vi "DAQ.vi"() -> ()   [LabVIEW 2014]
uses:
  <vilib>/express/express analysis/Spectral/Block/exnSpectralBlock spectral measurements PSD poly.vi
  <vilib>/express/express analysis/Spectral/Block/exnSpectralBlock spectral measurements PSD DDT.vi
  <vilib>/express/express analysis/Spectral/XNode/ExpressSpectralMeasurementsBlockNode.xnode
panel:
  out "Filtered PSD plot":dynamicdata(graph)
  out "RAW PSD plot":dynamicdata(graph)
  out "RAW & filtered Plot":dynamicdata(graph) caption="data"
  in  "File Comment":string caption="Comment"
  in  "Stop Daq":bool
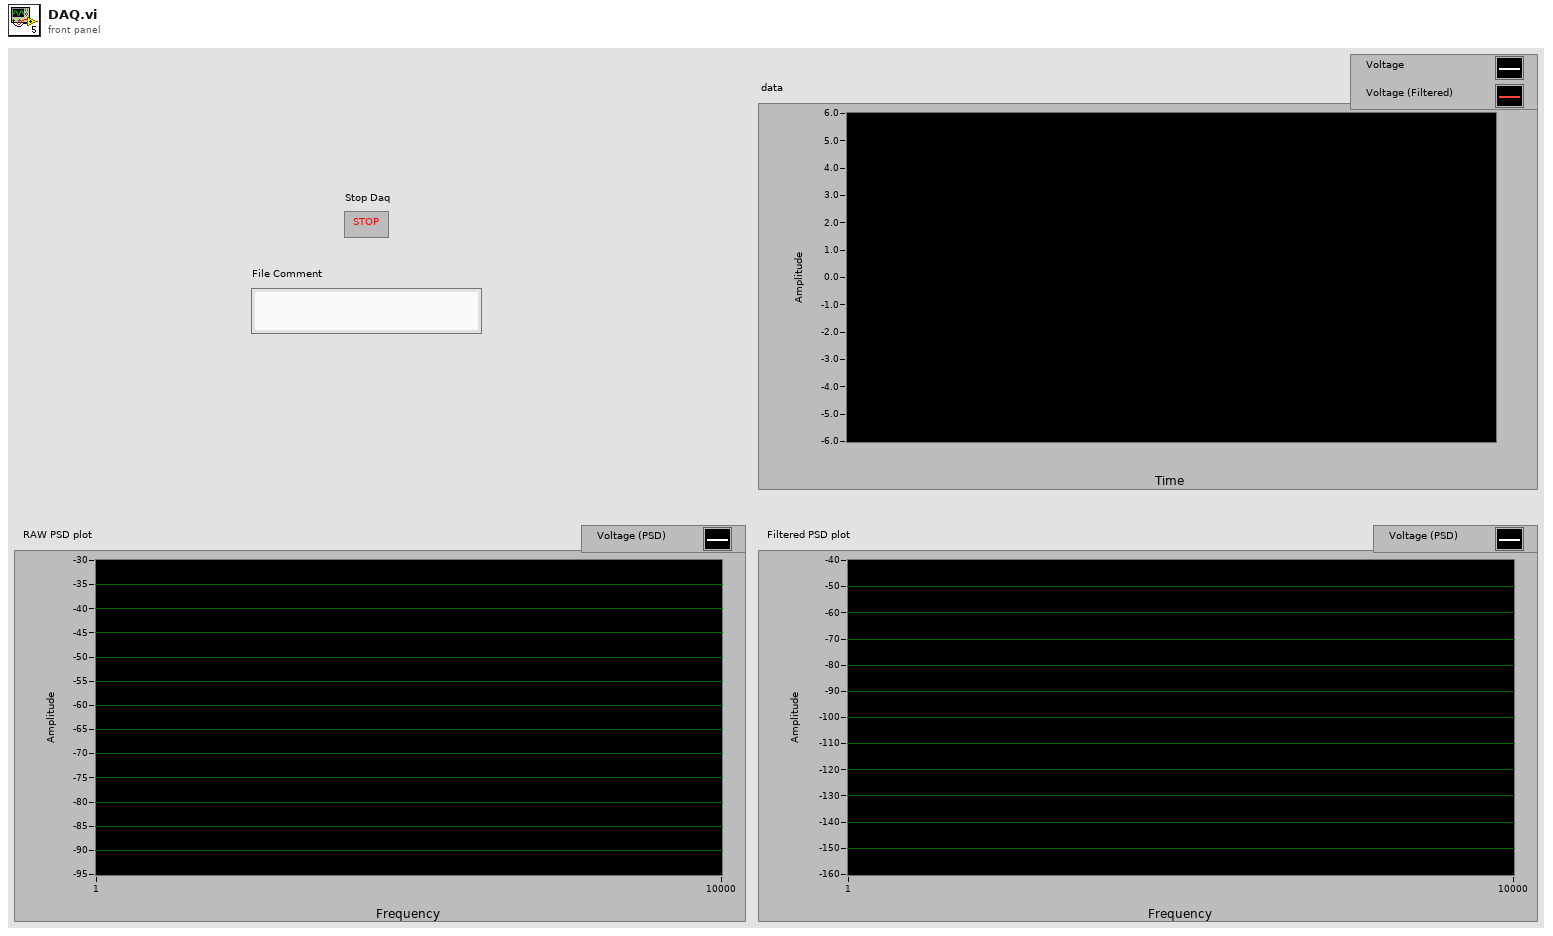
[diagram p1: front panel]
types:
  T1 = cluster{"averaging mode":u16, "weighting mode":u16, "number of averages":u32}
  T2 = cluster{"dB On (F)":bool, "unwrap phase (F)":bool, "convert to degree (F)":bool}
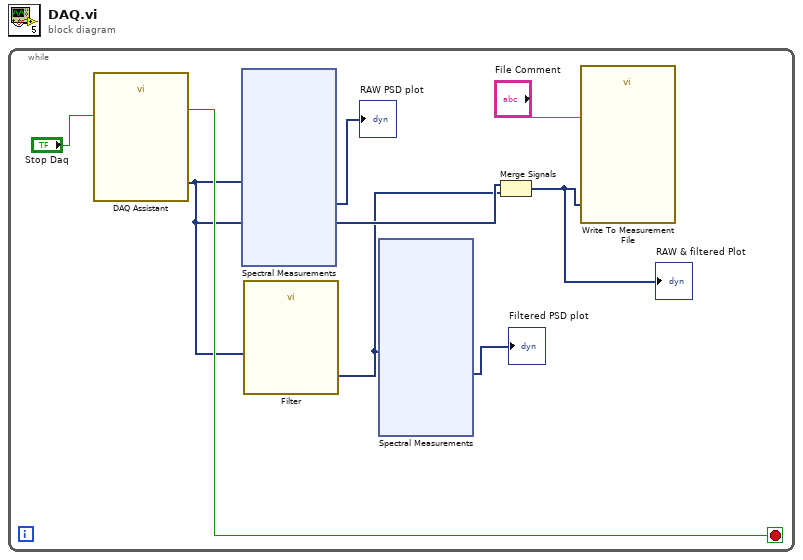
[diagram p0: block diagram]
diagram:
  n1 = while {
    stop <- w6 stop-if-true
    n2 = call "DAQ Assistant"("stop (F)"="Stop Daq") -> ("data"=w4:dynamicdata, "stopped"=w6:bool)  [unwired: 15 in, 2 out]
    n3 = xnode "Spectral Measurements"("Signals"=w4) -> ("PSD"=→"RAW PSD plot":dynamicdata)  [unwired: 2 in, 2 out]
    n4 = call "Filter"("Signal"=w4) -> ("Filtered Signal"=w2:dynamicdata)  [unwired: 9 in, 1 out]
    n5 = xnode "Spectral Measurements"("Signals"=w2) -> ("PSD"=→"Filtered PSD plot":dynamicdata)  [unwired: 2 in, 2 out]
    n6 = Merge Signals(w4, w2) -> (w5:dynamicdata)
    "RAW & filtered Plot" <- w5
    n7 = call "Write To Measurement File"("Signals"=w5, "Comment"="File Comment") -> ()  [unwired: 15 in, 3 out]
  }
